vi "Query_Keithley_Output.vi"(3 "error in (no error)":errorcluster, 5 "VISA resource name":refnum<visa-resource-name>) -> (0 "error out":errorcluster, 1 "Output":bool=TRUE, 2 "VISA resource name out":refnum<visa-resource-name>)   [LabVIEW 2015]
panel:
  out "Numeric":i32
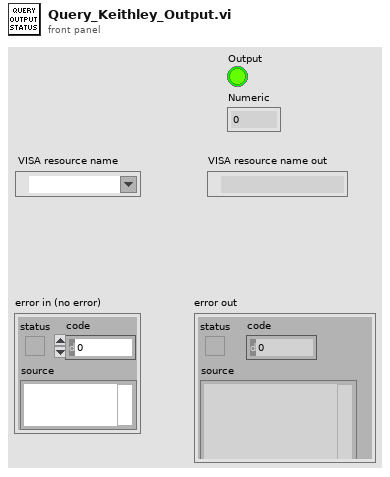
[diagram p1: front panel]
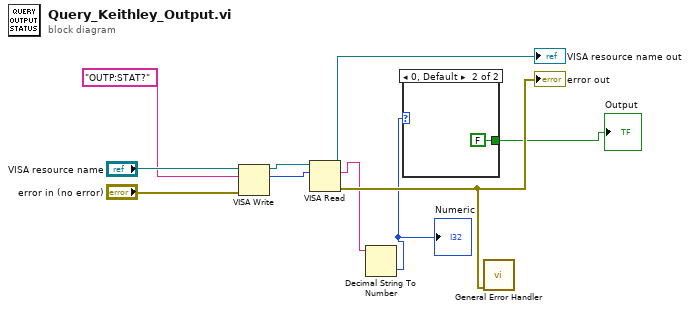
[diagram p0: block diagram]
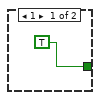
[diagram p2: hidden frame]
diagram:
  n1 = VISA Write(VISA resource name="VISA resource name", write buffer="OUTP:STAT?", error in (no error)="error in (no error)") -> (VISA resource name out=w7:refnum<visa-resource-name>, return count=w4:u32)  [unwired: 1 out]
  n2 = VISA Read(VISA resource name=w7, byte count=w4) -> (VISA resource name out=→"VISA resource name out":refnum<visa-resource-name>, read buffer=w2:string, error out=w5:errorcluster)  [unwired: 1 in, 1 out]
  "error out" <- w5
  n3 = Decimal String To Number(string=w2) -> (number=w1:i32)  [unwired: 2 in, 1 out]
  "Numeric" <- w1
  n4 = case shown="0, Default" w1 {
    tunnel: [TRUE FALSE] -> w3
    frame 1 {
    }
    frame 0, Default {
    }
  }
  "Output" <- w3
  n5 = call <vilib>:"General Error Handler.vi"("error in (no error)"=w5) -> ()  [unwired: 10 in, 5 out]
